vi "Voltage To Diode Write.vi"(8 "error in (no error)":errorcluster, 10 "Voltage":dbl, 11 "Top in":refnum<class "Top.lvclass">) -> (0 "error out":errorcluster, 3 "Top out":refnum<class "Top.lvclass">)   [LabVIEW 2021, in "Top.lvlib" / "Top.lvclass"]
uses:
  Top.lvclass
  Top.lvclass/Top.ctl
  <vilib>/NathanCo/Analog Tasks/Analog Output/Analog Output/Analog Output.lvclass
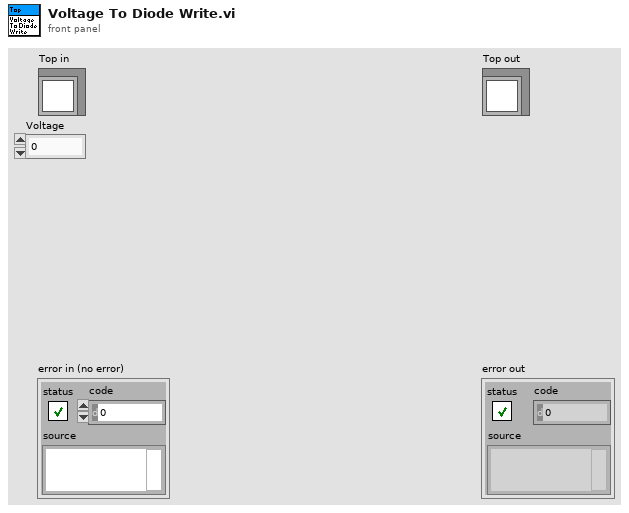
[diagram p1: front panel]
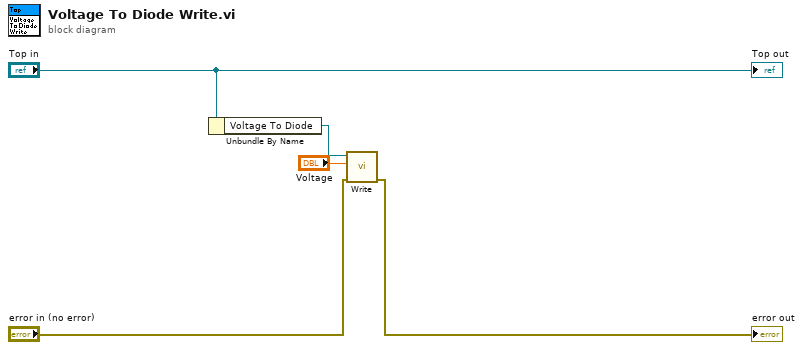
[diagram p0: block diagram]
diagram:
  n1 = Unbundle By Name("Top in") -> ("Voltage To Diode"=w4:refnum<class "Analog Output.lvclass">)
  n2 = call <vilib>:"Write.vi"("error in (no error)"="error in (no error)", "Voltage"="Voltage", "Analog Output in"=w4) -> ("error out"=→"error out":errorcluster)  [unwired: 8 in]
  "Top out" <- "Top in"
